vi "Write PGPASS.vi"(8 "error in":errorcluster, 11 "Connection Information":T1) -> (0 "error out":errorcluster)   [LabVIEW 2016, in "PQ Support.lvlib"]
uses:
  Connection Information.ctl
  <vilib>/Utility/sysdir.llb/System Directory Type.ctl
  PQ Support.lvlib
  Connection/PQ Connection.lvclass
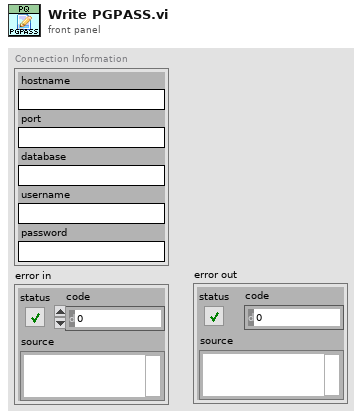
[diagram p1: front panel]
types:
  T1 = typedef "PQ Connection.lvclass/Connection Information.ctl" = cluster{"hostname":string, "port":string, "database":string, "username":string, "password":string}
  T2 = typedef "System Directory Type.ctl" = i32
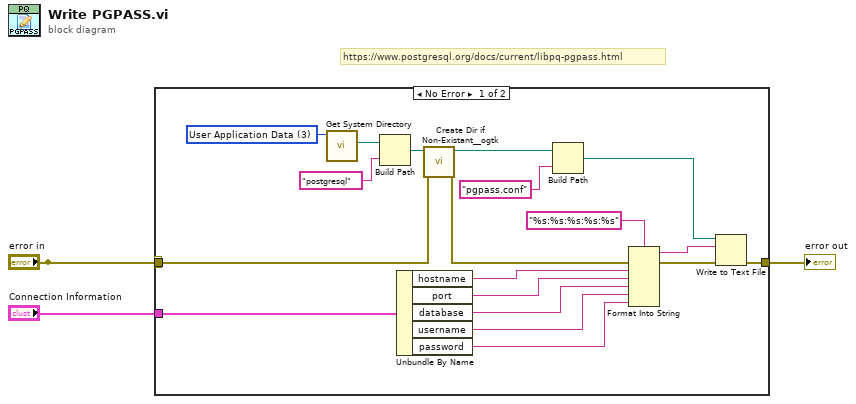
[diagram p0: block diagram]
diagram:
  # "https://www.postgresql.org/docs/current/libpq-pgpass.html"
  n1 = case shown="No Error" "error in" {
    selector: "error in" -> [_ w23]
    tunnel: [w12 w23] -> w3
    tunnel: "Connection Information" -> [w16 _]
    tunnel: "error in" -> [w5 _]
    frame No Error {
      w22 = T2 3 items=["User Home"=0, "User Desktop"=1, "User Documents"=2, "User Application Data"=3, "User Preferences"=4, "User Temporary"=5, "Public Documents"=6, "Public Application Data"=7, "Public Preferences"=8, "Public Cache"=13, "System Core Libraries"=9, "System Installed Libraries"=10, "Application Files"=11, "Boot Volume Root"=12] ("system directory type")
      n2 = call <vilib>:"Get System Directory.vi"("system directory type"=w22) -> ("system directory"=w21:path)  [unwired: 10 in]
      n3 = Build Path(base path=w21, name or relative path="postgresql") -> (appended path=w8:path)
      n4 = Unbundle By Name(w16) -> ("hostname"=w6:string, "port"=w9:string, "database"=w13:string, "username"=w14:string, "password"=w15:string)
      n5 = call <userlib>:"Create Dir if Non-Existant__ogtk.vi"("error in (no error)"=w5, "Directory Path"=w8) -> ("error out"=w4:errorcluster, "dup Directory Path"=w7:path)  [unwired: 7 in, 1 out]
      n6 = Build Path(base path=w7, name or relative path="pgpass.conf") -> (appended path=w10:path)
      n7 = Format Into String(format string="%s:%s:%s:%s:%s", error in=w4, w6, w9, w13, w14, w15) -> (resulting string=w17:string, error out=w11:errorcluster)  [unwired: 1 in]
      n8 = Write to Text File(file (use dialog)=w10, text=w17, error in=w11) -> (error out=w12:errorcluster)  [unwired: 1 in, 2 out]
    }
    frame Error {
    }
  }
  "error out" <- w3
